vi "Control Panel No Objects.vi"(8 "error in (no error)":errorcluster) -> (0 "error out":errorcluster)   [LabVIEW 2009]
doc: "(Dynamic) A user-level application that simulates the physical front panel of the Instrument. Provide the user with buttons to manually control features of the instrument, and provide indicators of its current state."
uses:
  Newport 1830-C/Public/Filters.ctl
  Global/GPIB Numbers.vi
panel:
  out "Initialized?":bool
  in  "Filter":T1=1 items=["Orange"=1, "Green"=2, "Yellow"=3]
  out "Power":string
  in  "Time between Reads (ms)":i32=200
  in  "Read Continuous":bool
  in  "Averaging Time (s)":dbl=0.5
  in  "Averaging":bool
  out "Units":u16(ring)=1 items=["W"=1, "dB"=2, "dBm"=3, "REL"=4]
  out "AVG":u16(ring)=2 items=["Slow"=1, "Medium"=2, "Fast"=3]
  out "Run/Stop":u16(ring) items=["Stop", "Run"]
  out "ATTN":u16(ring) items=["Off", "On"]
  out "Local Lockout":u16(ring) items=["Off", "On"]
  out "Zero":u16(ring) items=["Off", "On"]
  out "Beeper":u16(ring) items=["Off", "On"]
  out "Backlight":u16(ring) items=["Off", "Low", "High"]
  out "Range":u16(ring) items=["Auto", "Highest Sensitivity", "30uW", "300uW", "3mW", "30mW", "300mW", "3W", "Lowest Sensitivity"]
  in  "Run/Stop set":u32(ring)=1 items=["Stop", "Run"]
  in  "ATTN set":u32(ring) items=["Off", "On"]
  in  "BKLT set":u32(ring)=1 items=["Off", "Low", "High"]
  in  "Range set":u32(ring) items=["Auto", "Highest Sensitivity", "30uW", "300uW", "3mW", "30mW", "300mW", "3W", "Lowest Sensitivity"]
  in  "Beeper set":u32(ring) items=["Off", "On"]
  in  "AVG set":u32(ring)=2 items=["Slow"=1, "Medium"=2, "Fast"=3]
  in  "Units set":u32(ring)=1 items=["W"=1, "dB"=2, "mdB"=3, "REL"=4]
  in  "Zero set":u32(ring) items=["Off", "On"]
  in  "Local set":u32(ring) items=["Off", "On"]
  in  "Read Current Power":bool
  in  "Set":bool
  in  "Read to \nControl":bool
  in  "Read":bool
  in  "Wavelength Set":dbl[unit]
  out "Wavelength":dbl[unit]
  in  "Copy actual to set":bool
  in  "Populate fields with member data":bool
  in  "stop":bool
  # "With \nAttn\nOn"
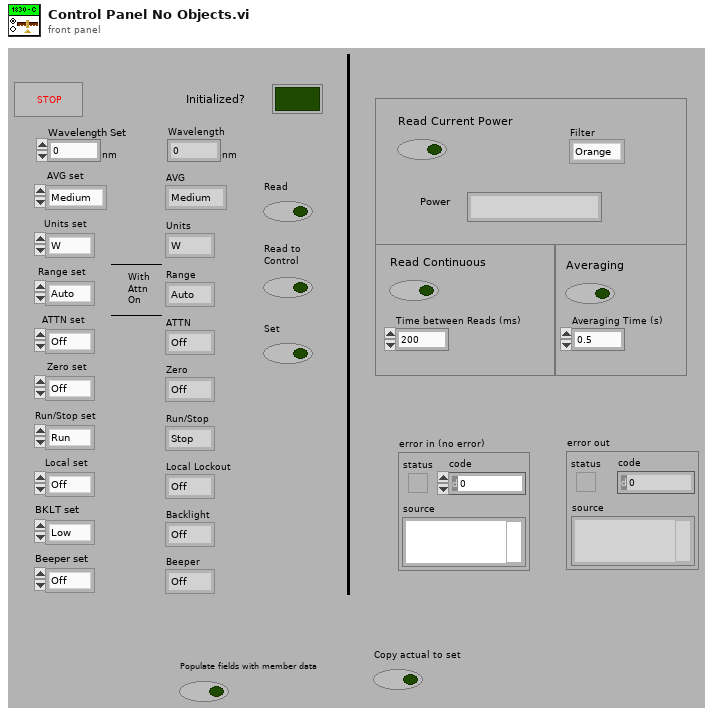
[diagram p1: front panel]
types:
  T1 = typedef "Filters.ctl" = u16
  T2 = cluster{"Wavelength":dbl[unit], "AVG":u16, "Range":u16, "Backlight":u16, "Beeper":u16, "Zero":u16, "Local Lockout":u16, "ATTN":u16, "Run/Stop":u16, "Units":u16, "Averaging Time":dbl, "Averaging":bool, "Most Recent Power":dbl, "Filter":T1}
  T3 = typedef "GPIB Type Def.ctl" = cluster{"Name":string, "bus":dbl, "GPIB":dbl, "GPIB as string":string, "byte":i32, "VISA Resource Name":refnum<visa-resource-name>}
  T4 = typedef "Readable.lvclass/X array.ctl" = T5[]
  T5 = typedef "Readable.lvclass/X.ctl" = dbl
  T6 = cluster{"Wavelength":dbl[unit], "AVG":i32, "Range":i32, "Backlight":i32, "Beeper":i32, "Zero":i32, "Local Lockout":i32, "ATTN":i32, "Run/Stop":i32, "Units":i32, "Averaging Time":dbl, "Averaging":bool, "Most Recent Power":dbl, "Filter":i32}
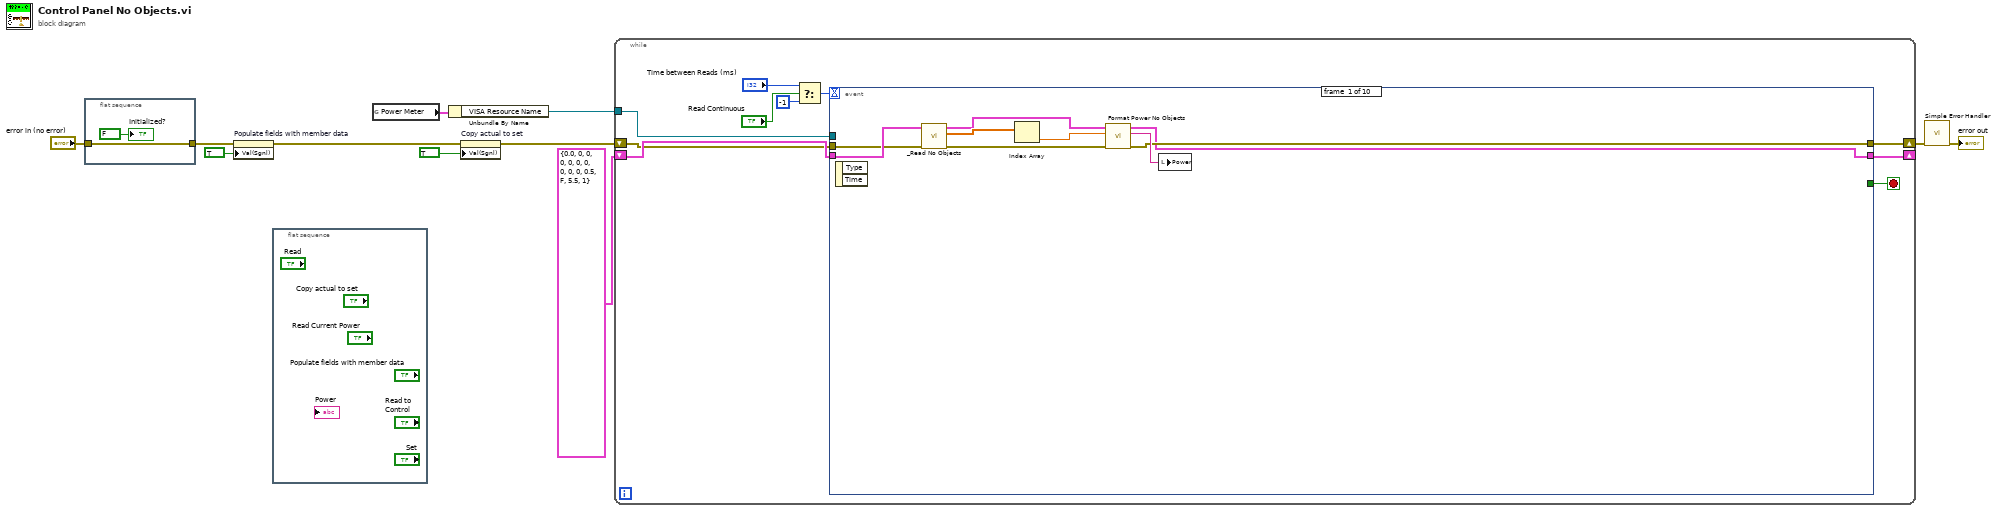
[diagram p0: block diagram]
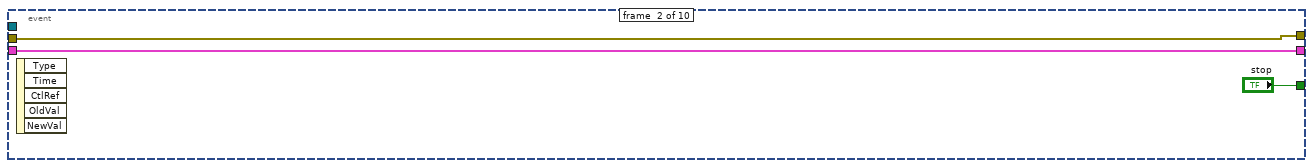
[diagram p2: hidden frame]
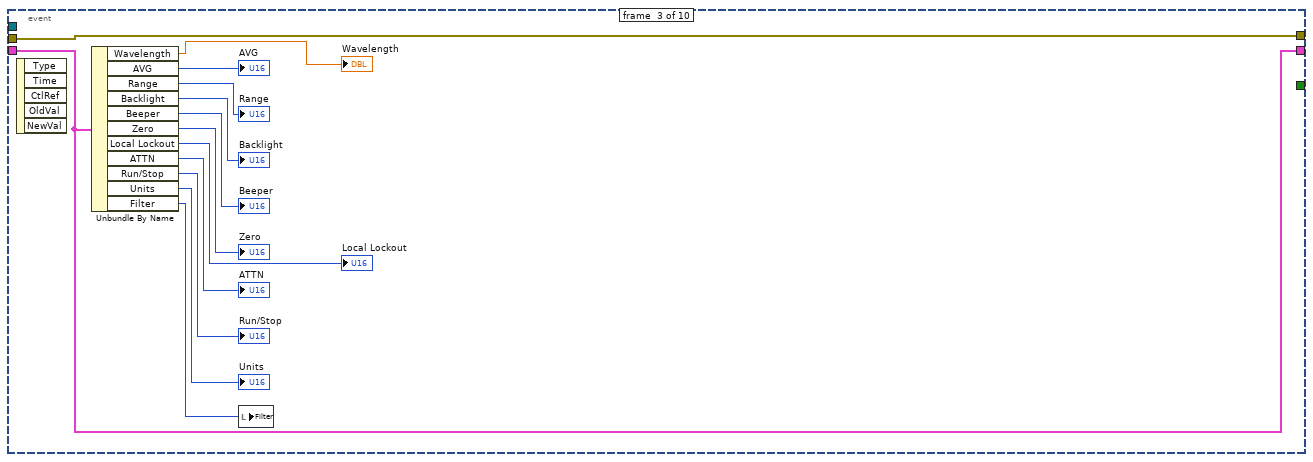
[diagram p3: hidden frame]
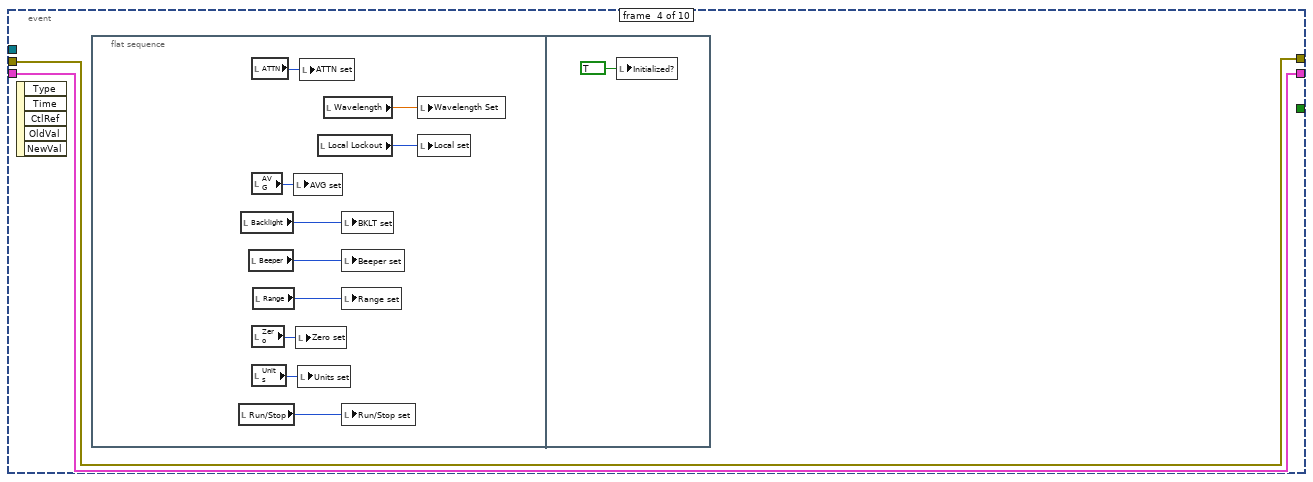
[diagram p4: hidden frame]
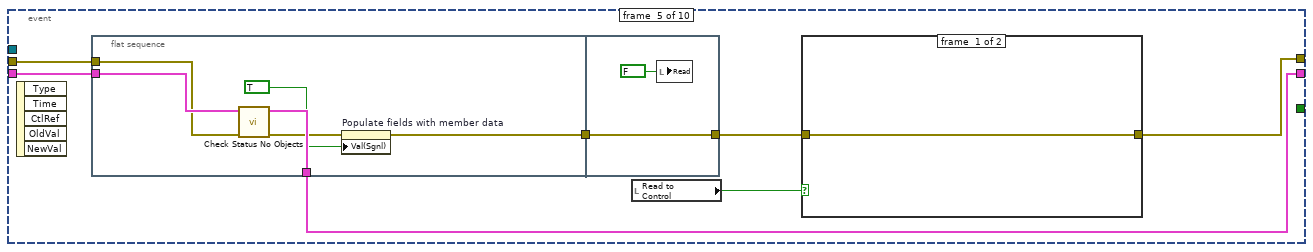
[diagram p5: hidden frame]
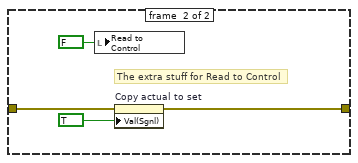
[diagram p6: hidden frame]
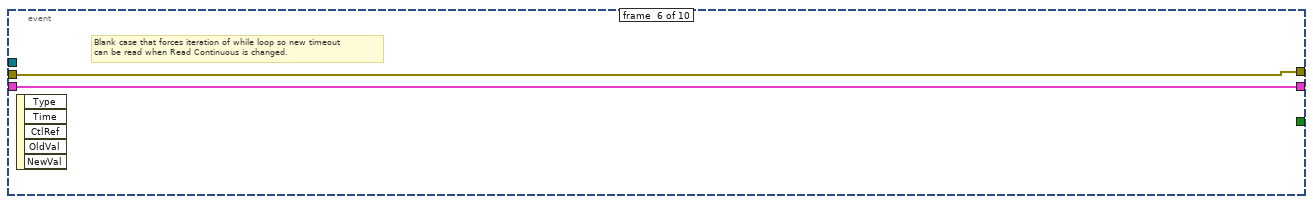
[diagram p7: hidden frame]
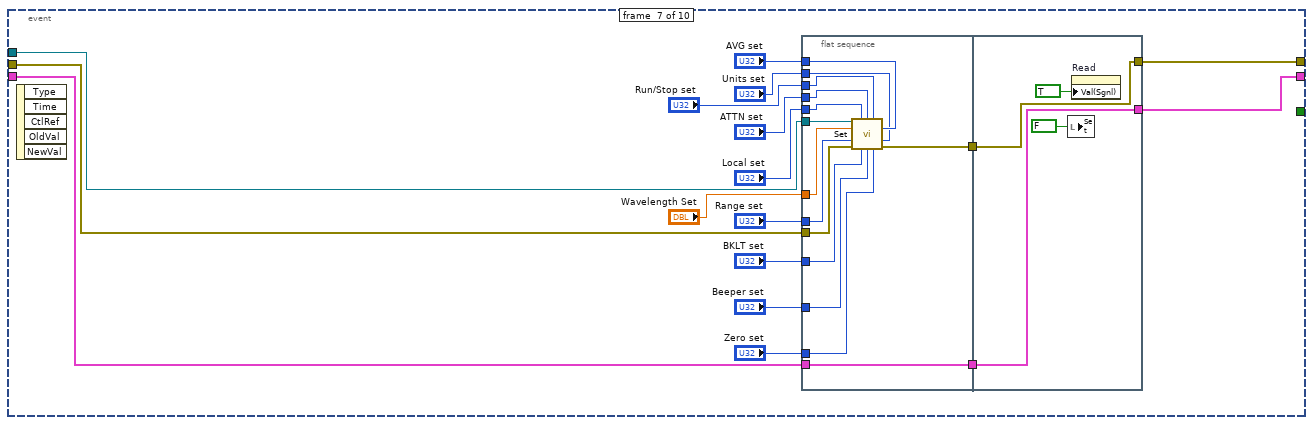
[diagram p8: hidden frame]
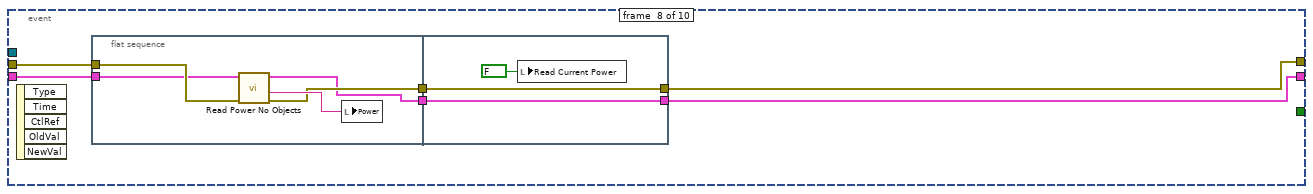
[diagram p9: hidden frame]
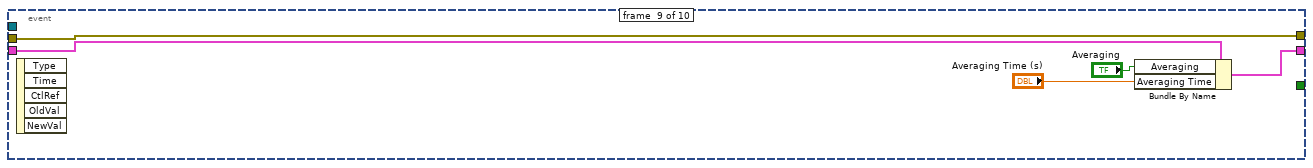
[diagram p10: hidden frame]
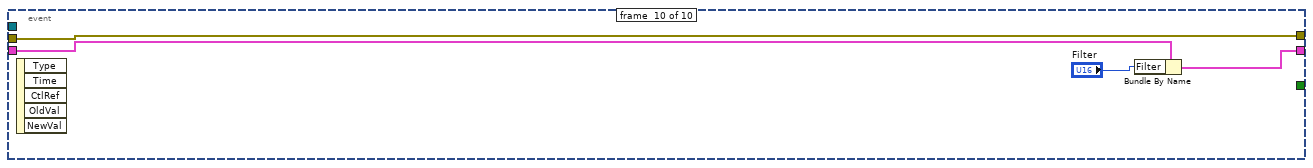
[diagram p11: hidden frame]
diagram:
  n1 = flat-sequence {
    tunnel: "error in (no error)" -> [w12]
    tunnel: [w12] -> w3
    frame #0 {
      "Initialized?" <- FALSE
    }
  }
  n2 = property on="Populate fields with member data" class="Bool (strict)"(error in=w3, "Val(Sgnl)"=TRUE ("Value (Signaling)")) -> (error out=w9:errorcluster)  [unwired: 1 in, 1 out]
  n3 = flat-sequence {
    frame #0 {
    }
  }
  n4 = global read "GPIB Numbers.vi" "Power Meter"() -> (w6:T3)
  n5 = Unbundle By Name(w6) -> ("VISA Resource Name"=w1:refnum<visa-resource-name>)
  n6 = property on="Copy actual to set" class="Bool (strict)"(error in=w9, "Val(Sgnl)"=TRUE ("Value (Signaling)")) -> (error out=w8:errorcluster)  [unwired: 1 in, 1 out]
  n7 = while {
    shift-right: [w20] -> _
    shift-left: T2 {"Wavelength"=0.0, "AVG"=0, "Range"=0, "Backlight"=0, "Beeper"=0, "Zero"=0, "Local Lockout"=0, "ATTN"=0, "Run/Stop"=0, "Units"=0, "Averaging Time"=0.5, "Averaging"=FALSE, "Most Recent Power"=5.5, "Filter"=1} ("Cluster of class private data") -> [w22]
    shift-right: [w19] -> w7
    shift-left: w8 -> [w21]
    tunnel: w1 -> [w14]
    stop <- w23 stop-if-true
    n8 = Select(t="Time between Reads (ms)", s="Read Continuous", f=-1) -> (s? t:f=w16:i32)
    n9 = event shown="[9] \"Filter\": Value Change" {
      selector: _ -> [_ _ _ _ _ _ _ _ _ _]
      dyn-events: _ -> [_ _ _ _ _ _ _ _ _ _]
      timeout: w16 -> [_ _ _ _ _ _ _ _ _ _]
      tunnel: [_ "stop" _ _ _ _ _ _ _ _] -> w23
      tunnel: [w25 w34 w47 w50 w62 w83 w97 w120 w136 w138] -> w20
      tunnel: w22 -> [w32 w34 w47 w50 w68 w83 w100 w124 w137 w141]
      tunnel: [w26 w33 w46 w49 w63 w82 w96 w119 w135 w139] -> w19
      tunnel: w21 -> [w31 w33 w46 w49 w67 w82 w98 w122 w135 w139]
      tunnel: w14 -> [_ _ _ _ _ _ w85 _ _ _]
      event #0 {
        n10 = event-data() -> ()  [unwired: 1 in, 2 out]
        n11 = call "_Read No Objects.vi"("error in (no error)"=w31, "Power Meter in"=w32) -> ("error out"=w30:errorcluster, "X array"=w29:T4, "Power Meter Out"=w24:T6)  [unwired: 7 in]
        n12 = Index Array(array=w29) -> (element=w28:T5)  [unwired: 1 in]
        n13 = call "Format Power No Objects.vi"("error in"=w30, "Power"=w28, "Cluster In"=w24) -> ("error out"=w26:errorcluster, "Formatted Power"=w27:string, "Cluster Out"=w25:T2)  [unwired: 6 in]
        n14 = local write "Power"(w27) -> ()
      }
      event #1 {
        n15 = event-data() -> ()  [unwired: 1 in, 5 out]
      }
      event #2 {
        n16 = event-data() -> ()  [unwired: 1 in, 5 out]
        n17 = Unbundle By Name(w47) -> ("Wavelength"=→"Wavelength":dbl[unit], "AVG"=→"AVG":i32, "Range"=→"Range":i32, "Backlight"=→"Backlight":i32, "Beeper"=→"Beeper":i32, "Zero"=→"Zero":i32, "Local Lockout"=→"Local Lockout":i32, "ATTN"=→"ATTN":i32, "Run/Stop"=→"Run/Stop":i32, "Units"=→"Units":i32, "Filter"=w36:i32)
        n18 = local write "Filter"(w36) -> ()
      }
      event #3 {
        n19 = event-data() -> ()  [unwired: 1 in, 5 out]
        n20 = flat-sequence {
          frame #0 {
            n21 = local read "Run/Stop"() -> (w54:u16)
            n22 = local read "Backlight"() -> (w58:u16)
            n23 = local read "Beeper"() -> (w57:u16)
            n24 = local read "ATTN"() -> (w52:u16)
            n25 = local read "AVG"() -> (w59:u16)
            n26 = local read "Zero"() -> (w51:u16)
            n27 = local read "Units"() -> (w53:u16)
            n28 = local read "Range"() -> (w55:u16)
            n29 = local write "AVG set"(w59) -> ()
            n30 = local write "Zero set"(w51) -> ()
            n31 = local write "Units set"(w53) -> ()
            n32 = local write "ATTN set"(w52) -> ()
            n33 = local read "Local Lockout"() -> (w56:u16)
            n34 = local read "Wavelength"() -> (w60:dbl[unit])
            n35 = local write "BKLT set"(w58) -> ()
            n36 = local write "Beeper set"(w57) -> ()
            n37 = local write "Range set"(w55) -> ()
            n38 = local write "Run/Stop set"(w54) -> ()
            n39 = local write "Wavelength Set"(w60) -> ()
            n40 = local write "Local set"(w56) -> ()
          }
          frame #1 {
            n41 = local write "Initialized?"(TRUE ("Power\nMeter\nInitialized?")) -> ()
          }
        }
      }
      event #4 {
        n42 = event-data() -> ()  [unwired: 1 in, 5 out]
        n43 = flat-sequence {
          tunnel: w68 -> [w79]
          tunnel: w67 -> [w78]
          tunnel: [w75] -> w64
          tunnel: [w77] -> w62
          tunnel: [w80] -> w65
          tunnel: w64 -> [w80]
          frame #0 {
            n44 = call "Check Status No Objects.vi"("error in (no error)"=w78, "Power Meter in"=w79) -> ("error out"=w76:errorcluster, "Power Meter out"=w77:T6)  [unwired: 6 in, 1 out]
            n45 = property on="Populate fields with member data" class="Bool (strict)"(error in=w76, "Val(Sgnl)"=TRUE ("Value (Signaling)")) -> (error out=w75:errorcluster)  [unwired: 1 in, 1 out]
          }
          frame #1 {
            n46 = local write "Read"(FALSE ("Read")) -> ()
          }
        }
        n47 = local read "Read to \nControl"() -> (w66:bool)
        n48 = case shown="True" w66 {
          tunnel: w65 -> [w69 w71]
          tunnel: [w69 w70] -> w63
          frame #0 {
          }
          frame #1 {
            # "The extra stuff for Read to Control"
            n49 = local write "Read to \nControl"(FALSE ("Read")) -> ()
            n50 = property on="Copy actual to set" class="Bool (strict)"(error in=w71, "Val(Sgnl)"=TRUE ("Value (Signaling)")) -> (error out=w70:errorcluster)  [unwired: 1 in, 1 out]
          }
        }
      }
      event #5 {
        # "Blank case that forces iteration of while loop so new timeout\ncan be read when Read Continuous is changed."
        n51 = event-data() -> ()  [unwired: 1 in, 5 out]
      }
      event #6 {
        n52 = event-data() -> ()  [unwired: 1 in, 5 out]
        n53 = flat-sequence {
          tunnel: w100 -> [w103]
          tunnel: [w102] -> w99
          tunnel: w98 -> [w101]
          tunnel: "AVG set" -> [w114]
          tunnel: "Units set" -> [w113]
          tunnel: "Run/Stop set" -> [w112]
          tunnel: "ATTN set" -> [w111]
          tunnel: "Local set" -> [w110]
          tunnel: "Wavelength Set" -> [w109]
          tunnel: "Range set" -> [w108]
          tunnel: "BKLT set" -> [w107]
          tunnel: "Beeper set" -> [w106]
          tunnel: "Zero set" -> [w105]
          tunnel: w85 -> [w104]
          tunnel: [w103] -> w84
          tunnel: [w115] -> w97
          tunnel: [w116] -> w96
          tunnel: w99 -> [w116]
          tunnel: w84 -> [w115]
          frame #0 {
            n54 = call "Set.vi"("VISA resource name"=w104, "Local Lockout (0:1)"=w110, "ATTN (0:1)"=w111, "Run/Stop (1:0)"=w112, "Wavelength (nnnn)"=w109, "AVG (1:3)"=w114, "Range (0-Auto,1:8)"=w108, "Units (1:4)"=w113, "error in (no error)"=w101, "Backlight (0:2)"=w107, "Beeper (0:1)"=w106, "Zero (0:1)"=w105) -> ("error out"=w102:errorcluster)  [unwired: 2 in, 1 out]
          }
          frame #1 {
            n55 = local write "Set"(FALSE ("Set")) -> ()
            n56 = property on="Read" class="Bool (strict)"("Val(Sgnl)"=TRUE ("Value (Signaling)")) -> ()  [unwired: 2 in, 2 out]
          }
        }
      }
      event #7 {
        n57 = event-data() -> ()  [unwired: 1 in, 5 out]
        n58 = flat-sequence {
          tunnel: w124 -> [w125]
          tunnel: [w126] -> w123
          tunnel: w122 -> [w129]
          tunnel: [w127] -> w121
          tunnel: [w131] -> w120
          tunnel: w123 -> [w131]
          tunnel: [w130] -> w119
          tunnel: w121 -> [w130]
          frame #0 {
            n59 = call "Read Power No Objects.vi"("error in (no error)"=w129, "Cluster In"=w125) -> ("error out"=w127:errorcluster, "Current Power w/ Units"=w128:string, "Cluster Out"=w126:T2)  [unwired: 6 in, 1 out]
            n60 = local write "Power"(w128) -> ()
          }
          frame #1 {
            n61 = local write "Read Current Power"(FALSE ("Read Current Value")) -> ()
          }
        }
      }
      event #8 {
        n62 = event-data() -> ()  [unwired: 1 in, 5 out]
        n63 = Bundle By Name(cluster=w137, "Averaging"="Averaging", "Averaging Time"="Averaging Time (s)") -> (w136:T6)
      }
      event #9 {
        n64 = event-data() -> ()  [unwired: 1 in, 5 out]
        n65 = Bundle By Name(cluster=w141, "Filter"="Filter") -> (w138:T6)
      }
    }
  }
  n66 = call <vilib>:"Simple Error Handler.vi"("error in (no error)"=w7) -> ("error out"=→"error out":errorcluster)  [unwired: 1 in, 7 out]
